vi "Library New File.vi"(6 "overwrite (F)":bool, 8 "error in (no error)":errorcluster, 9 "deny mode (deny none)":T1(ring)=enum."deny none", 11 "file path":path) -> (0 "error out":errorcluster, 3 "refnum":refnum<file>)   [LabVIEW 2012]
doc: "This is a drop-in replacement for the LabVIEW \"new file\" node with as only enhancement less useless error reporting through showing the path of the file that could not be opened as part of the error message."
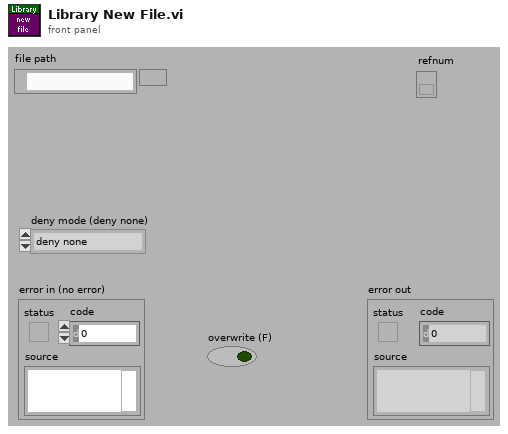
[diagram p1: front panel]
types:
  T1 = enum16{"deny read/write", "deny write-only", "deny none"}
  T2 = enum16{"open", "replace", "create", "open or create", "replace or create", "replace or create with confirmation"}
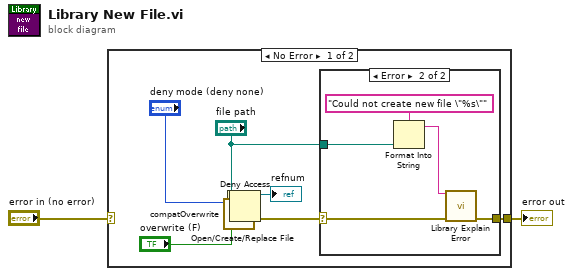
[diagram p0: block diagram]
diagram:
  n1 = case shown="No Error" "error in (no error)" {
    selector: "error in (no error)" -> [_ w18]
    tunnel: [w8 w18] -> w2
    frame No Error {
      n2 = call <vilib>:"compatOverwrite.vi"("overwrite (F)"="overwrite (F)") -> ("overwrite?"=w3:T2)
      n3 = Open/Create/Replace File(file path (use dialog)="file path", operation (0:open)=w3) -> (refnum out=w4:refnum<file>, error out=w5:errorcluster)  [unwired: 4 in, 1 out]
      n4 = Deny Access(4:w5, 6:"deny mode (deny none)", 7:w4) -> (0:w9:errorcluster, 3:→"refnum":refnum<file>)
      n5 = case shown="Error" w9 {
        selector: w9 -> [w12 w13]
        tunnel: "file path" -> [_ w17]
        tunnel: [w12 w14] -> w8
        frame No Error {
        }
        frame Error {
          n6 = Format Into String(format string="Could not create new file \"%s\"", w17) -> (resulting string=w15:string)  [unwired: 2 in, 1 out]
          n7 = call "Library Explain Error.vi"("explanation prefix (none)"=w15, "error in (no error)"=w13) -> ("explained error"=w14:errorcluster)  [unwired: 13 in]
        }
      }
    }
    frame Error {
    }
  }
  "error out" <- w2
